vi "Request Channel.vi"(0 "Display State In":T2={"Hierarchy"=[], "File/Directory Path"=path "", "Relative File Paths"=[], "Hide Undefined Channels"=FALSE, "Static File Structure"=FALSE, "Filtering"={"Filtered Groups"=[], "Group Filter Mode"=enum."Exclude", "Group Filter Regex?"=FALSE, "Filtered Channels"=[], "Channel Filter Mode"=enum."Exclude", "Channel Filter Regex?"=FALSE, "Filter Time Start"=timestamp(0 s since 1904-01-01), "Filter Time End"=timestamp(0 s since 1904-01-01), "Time Filter Mode"=enum."Include", "Time Filter Enabled"=FALSE}, "File Contents Tree"=refnum, "Properties Table"=refnum, "Loading Indicator"=refnum}, 1 "Use Regular Expressions?":bool, 5 "Group Name":string, 7 "Channel Name":string, 9 "Container State":T5, 11 "error in (no error)":errorcluster) -> (4 "Display State Out":T2={"Hierarchy"=[], "File/Directory Path"=path "", "Relative File Paths"=[], "Hide Undefined Channels"=FALSE, "Static File Structure"=FALSE, "Filtering"={"Filtered Groups"=[], "Group Filter Mode"=enum."Exclude", "Group Filter Regex?"=FALSE, "Filtered Channels"=[], "Channel Filter Mode"=enum."Exclude", "Channel Filter Regex?"=FALSE, "Filter Time Start"=timestamp(0 s since 1904-01-01), "Filter Time End"=timestamp(0 s since 1904-01-01), "Time Filter Mode"=enum."Include", "Time Filter Enabled"=FALSE}, "File Contents Tree"=refnum, "Properties Table"=refnum, "Loading Indicator"=refnum}, 6 "Channel Data":T1[](array[typedef]), 15 "error out":errorcluster)   [LabVIEW 2017, in "XTree.xctl"]
doc: "Request one or more channels from the files currently represented in the tree. The Group Name and Channel Name inputs support regular expressions."
uses:
  <vilib>/addons/_NIFileIO/XTree/XTree.xctl
  <vilib>/_xctls/Container State.ctl
  <vilib>/addons/_NIFileIO/XTree/State.ctl
  <vilib>/addons/_NIFileIO/XTree/Controls/Filter Settings.ctl
  <vilib>/addons/_NIFileIO/XTree/Controls/Filter Mode.ctl
  <vilib>/addons/_NIFileIO/XTree/Controls/Tree Selection Data.ctl
  <vilib>/_xctls/XControlSupport.lvlib
panel:
  # "Add Controls & Indicators that form the parameters of the method here. Hook them to the connector pane. Do not delete the controls & indicators that are already hooked to the connector pane.\n \nTo setup the parameters  for this method, right click on this item in the Project Tree & select \"Configure Method...\"."
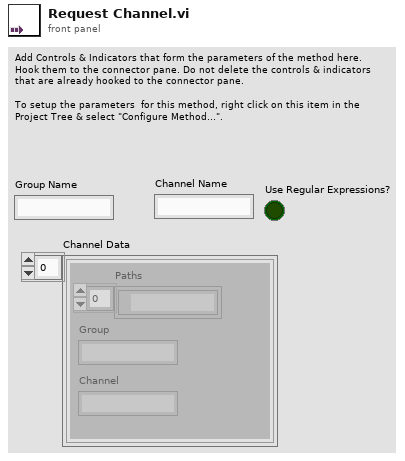
[diagram p1: front panel]
types:
  T1 = typedef "XTree.xctl/Tree Selection Data.ctl" = cluster{"Paths":path[], "Group":string, "Channel":string}
  T2 = typedef "XTree.xctl/State.ctl" = cluster{"Hierarchy":string[], "File/Directory Path":path, "Relative File Paths":string[], "Hide Undefined Channels":bool, "Static File Structure":bool, "Filtering":T3, "File Contents Tree":refnum<vi>, "Properties Table":refnum<vi>, "Loading Indicator":refnum<vi>}
  T3 = typedef "XTree.xctl/Filter Settings.ctl" = cluster{"Filtered Groups":string[], "Group Filter Mode":T4, "Group Filter Regex?":bool, "Filtered Channels":string[], "Channel Filter Mode":T4, "Channel Filter Regex?":bool, "Filter Time Start":timestamp, "Filter Time End":timestamp, "Time Filter Mode":T4, "Time Filter Enabled":bool}
  T4 = typedef "XTree.xctl/Filter Mode.ctl" = enum16{"Exclude", "Include"}
  T5 = typedef "XControlSupport.lvlib/Container State.ctl" = cluster{"Indicator?":bool, "Run Mode?":bool, " Refnum":refnum<vi>}
  T6 = enum16{"open", "open or create", "create or replace", "create", "open (read-only)"}
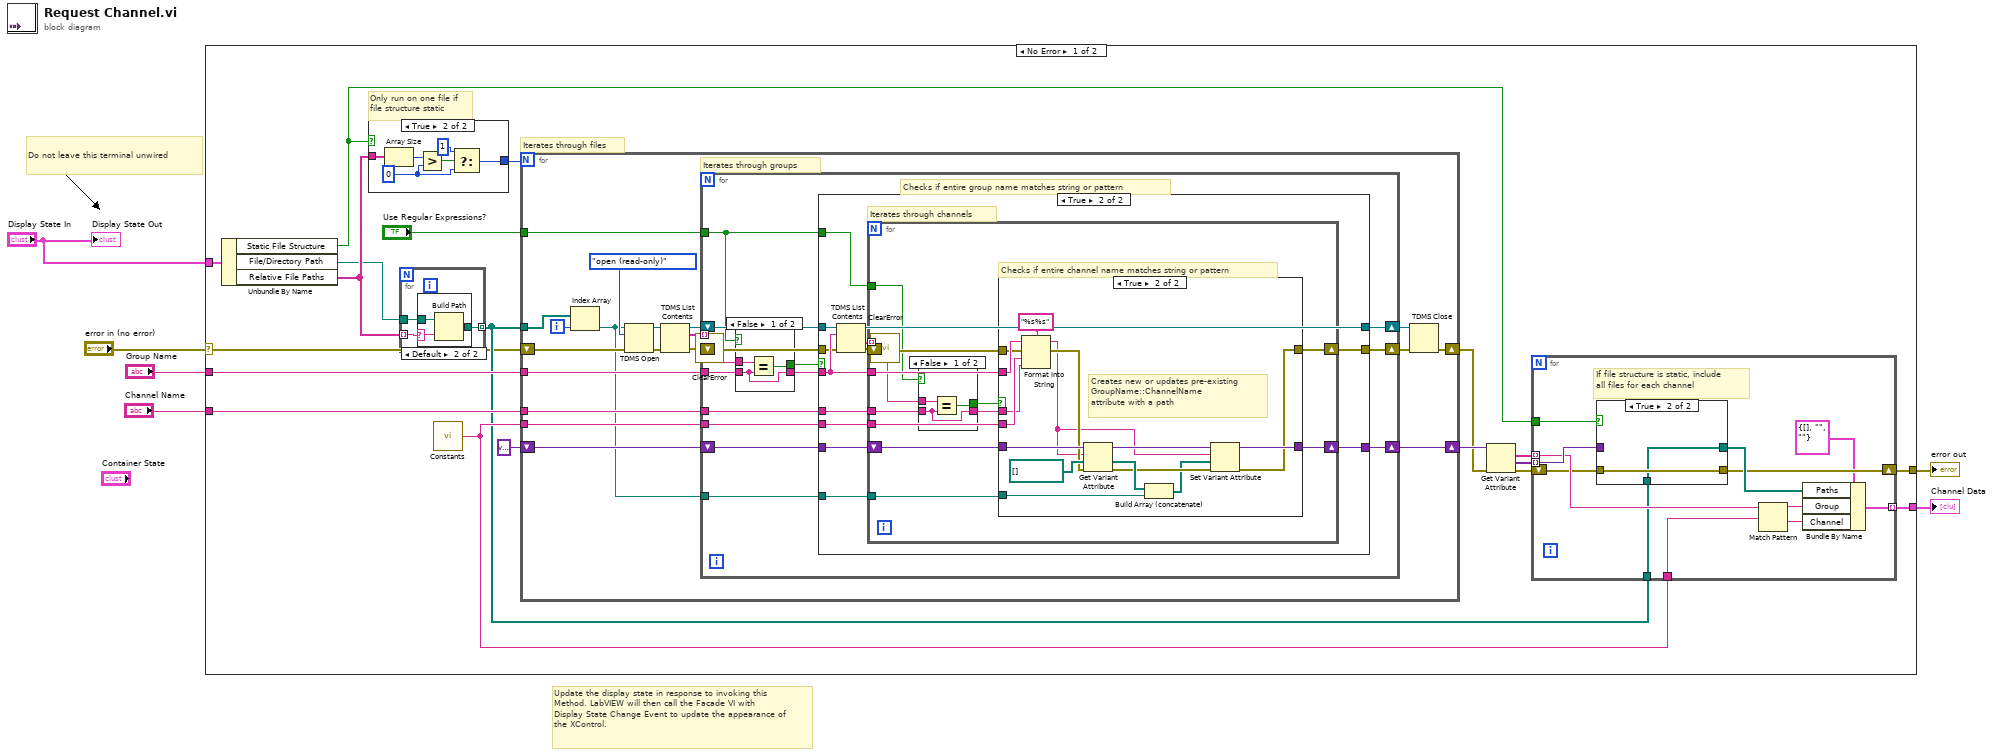
[diagram p0: block diagram]
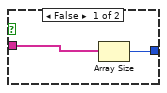
[diagram p3: hidden frame]
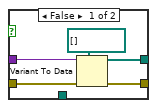
[diagram p4: hidden frame]
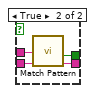
[diagram p5: hidden frame]
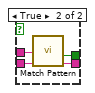
[diagram p7: hidden frame]
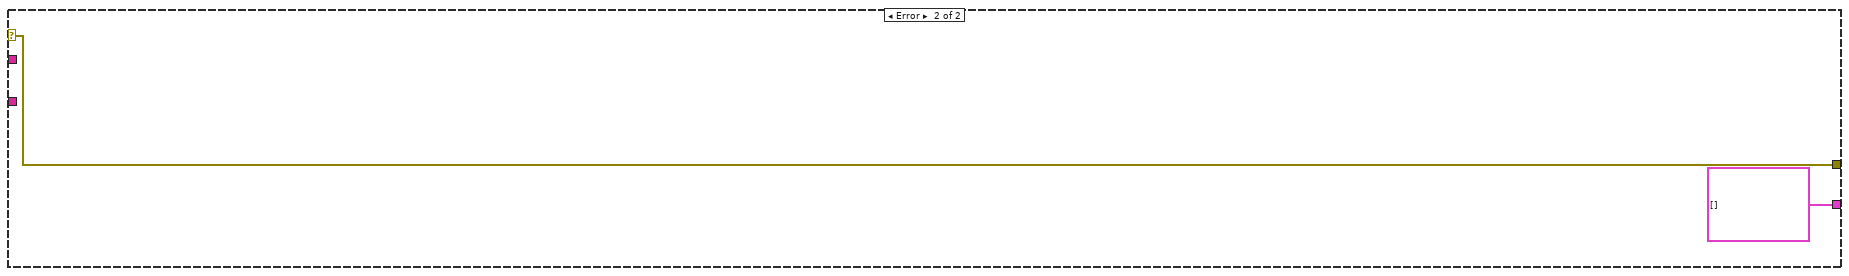
[diagram p9: hidden frame]
diagram:
  # "Do not leave this terminal unwired"
  # "Update the display state in response to invoking this Method. LabVIEW will then call the Facade VI with Display State Change Event to update the appearance of the XControl."
  n1 = case shown="No Error" "error in (no error)" {
    selector: "error in (no error)" -> [w7 w156]
    tunnel: "Display State In" -> [w25 _]
    tunnel: "Group Name" -> [w24 _]
    tunnel: "Channel Name" -> [w23 _]
    tunnel: [w17 T1[] []] -> w3
    tunnel: [w13 w156] -> w2
    frame No Error {
      # "Iterates through files"
      # "Only run on one file if file structure static"
      n2 = Unbundle By Name(w25) -> ("Static File Structure"=w12:bool, "File/Directory Path"=w8:path, "Relative File Paths"=w11:string[])
      n3 = case shown="True" w12 {
        tunnel: [w34 w35] -> w15
        tunnel: w11 -> [w33 w40]
        frame False {
          n4 = Array Size(array=w33) -> (size(s)=w34:i32)
        }
        frame True {
          w37 = 0 ("y")
          n5 = Array Size(array=w40) -> (size(s)=w39:i32)
          n6 = Greater?(x=w39, y=w37) -> (0:w38:bool)
          n7 = Select(t=1, s=w38, f=w37) -> (s? t:f=w35:i32)
        }
      }
      n8 = for {
        tunnel: w11 -> [w26] mode=indexing
        tunnel: w8 -> [w28]
        tunnel: [w27] -> w10 mode=indexing
        n9 = case shown="Default" w26 {
          selector: w26 -> [_ w30]
          tunnel: w28 -> [w29 w32]
          tunnel: [w29 w31] -> w27
          frame "" {
          }
          frame Default {
            n10 = Build Path(base path=w32, name or relative path=w30) -> (appended path=w31:path)
          }
        }
      }
      n11 = call <vilib>:"Constants.vi"() -> ("String Delimeter"=w16:string)  [unwired: 5 in]
      n12 = for {
        N: w15 -> [_]
        shift-right: [w79] -> w20
        shift-left: w7 -> [w65]
        tunnel: w24 -> [w74]
        tunnel: w23 -> [w72]
        tunnel: w16 -> [w67]
        shift-right: [w66] -> w21
        shift-left: variant ("variant") -> [w68]
        tunnel: w10 -> [w63]
        tunnel: "Use Regular Expressions?" -> [w64]
        i -> [w61]
        # "Iterates through groups"
        n13 = Index Array(array=w63, index=w61) -> (element=w62:path)
        n14 = TDMS Open(8:w65, 10:T6."open (read-only)" ("operation (0:open)"), 11:w62) -> (0:w77:errorcluster, 3:w76:refnum<k34>)  [unwired: 4 in]
        n15 = TDMS List Contents(4:w77, 7:w76) -> (0:w60:errorcluster, 2:w75:string[], 3:w73:refnum<k34>)  [unwired: 1 in, 1 out]
        n16 = call <vilib>:"ClearError.vi"("error in (no error)"=w60) -> ("error out"=w70:errorcluster)
        n17 = for {
          tunnel: w75 -> [w93] mode=indexing
          tunnel: w74 -> [w91]
          tunnel: w72 -> [w89]
          shift-right: [w88] -> w71
          shift-left: w73 -> [w92]
          shift-right: [w87] -> w69
          shift-left: w70 -> [w82]
          tunnel: w67 -> [w85]
          tunnel: w62 -> [w84]
          shift-right: [w83] -> w66
          shift-left: w68 -> [w86]
          tunnel: w64 -> [w80]
          # "Checks if entire group name matches string or pattern"
          n18 = case shown="False" w80 {
            tunnel: w93 -> [w96 w98]
            tunnel: w91 -> [w94 w100]
            tunnel: [w94 w99] -> w90
            tunnel: [w95 w97] -> w81
            frame False {
              n19 = Equal?(x=w96, y=w94) -> (x = y?=w95:bool)
            }
            frame True {
              n20 = call <vilib>:"Match Pattern.vi"("Pattern"=w100, "String in"=w98) -> ("String out"=w99:string, "Match?"=w97:bool)  [unwired: 8 in]
            }
          }
          n21 = case shown="True" w81 {
            tunnel: w90 -> [_ w114]
            tunnel: w92 -> [w103 w117]
            tunnel: w89 -> [_ w115]
            tunnel: [w103 w113] -> w88
            tunnel: w82 -> [w102 w112]
            tunnel: [w102 w110] -> w87
            tunnel: w86 -> [w101 w109]
            tunnel: w85 -> [_ w108]
            tunnel: w84 -> [_ w107]
            tunnel: [w101 w106] -> w83
            tunnel: w80 -> [_ w105]
            frame False {
            }
            frame True {
              # "Iterates through channels"
              n22 = TDMS List Contents(4:w112, 6:w114, 7:w117) -> (0:w104:errorcluster, 1:w116:string[], 3:w113:refnum<k34>)  [unwired: 1 out]
              n23 = call <vilib>:"ClearError.vi"("error in (no error)"=w104) -> ("error out"=w111:errorcluster)
              n24 = for {
                tunnel: w116 -> [w121] mode=indexing
                tunnel: w115 -> [w120]
                tunnel: w114 -> [w129]
                shift-right: [w128] -> w110
                shift-left: w111 -> [w123]
                tunnel: w108 -> [w126]
                tunnel: w107 -> [w125]
                shift-right: [w124] -> w106
                shift-left: w109 -> [w127]
                tunnel: w105 -> [w122]
                # "Checks if entire channel name matches string or pattern"
                n25 = case shown="False" w122 {
                  tunnel: w121 -> [w132 w134]
                  tunnel: w120 -> [w130 w136]
                  tunnel: [w130 w135] -> w118
                  tunnel: [w131 w133] -> w119
                  frame False {
                    n26 = Equal?(x=w132, y=w130) -> (x = y?=w131:bool)
                  }
                  frame True {
                    n27 = call <vilib>:"Match Pattern.vi"("Pattern"=w136, "String in"=w134) -> ("String out"=w135:string, "Match?"=w133:bool)  [unwired: 8 in]
                  }
                }
                n28 = case shown="True" w119 {
                  tunnel: w129 -> [_ w152]
                  tunnel: w123 -> [w138 w151]
                  tunnel: [w138 w142] -> w128
                  tunnel: w127 -> [w137 w154]
                  tunnel: w126 -> [_ w153]
                  tunnel: w125 -> [_ w144]
                  tunnel: [w137 w143] -> w124
                  tunnel: w118 -> [_ w139]
                  frame False {
                  }
                  frame True {
                    # "Creates new or updates pre-existing\nGroupName::ChannelName\nattribute with a path"
                    n29 = Format Into String(format string="%s%s", initial string=w152, error in=w151, w153, w139) -> (resulting string=w145:string, error out=w149:errorcluster)
                    n30 = Get Variant Attribute(Variant=w154, name=w145, default value (empty Variant)=path[] [], error in=w149) -> (duplicate Variant=w148:variant, value=w147:path[], error out=w146:errorcluster)  [unwired: 1 out]
                    n31 = Build Array (concatenate)(w147, w144) -> (w140:path[])
                    n32 = Set Variant Attribute(Variant=w148, name=w145, value=w140, error in=w146) -> (Variant out=w143:variant, error out=w142:errorcluster)  [unwired: 1 out]
                  }
                }
              }
            }
          }
        }
        n33 = TDMS Close(8:w69, 11:w71) -> (0:w79:errorcluster)  [unwired: 1 out]
      }
      n34 = Get Variant Attribute(Variant=w21, error in=w20) -> (names=w19:string[], values=w18:variant[], error out=w14:errorcluster)  [unwired: 2 in, 1 out]
      n35 = for {
        tunnel: w19 -> [w48] mode=indexing
        tunnel: w18 -> [w52] mode=indexing
        tunnel: [w47] -> w17 mode=indexing
        tunnel: w16 -> [w46]
        tunnel: w12 -> [w45]
        shift-right: [w43] -> w13
        shift-left: w14 -> [w44]
        tunnel: w10 -> [w42]
        # "If file structure is static, include all files for each channel"
        n36 = case shown="True" w45 {
          tunnel: w52 -> [w53 _]
          tunnel: [w56 w58] -> w51
          tunnel: w44 -> [w55 w59]
          tunnel: [w54 w59] -> w43
          tunnel: w42 -> [_ w58]
          frame False {
            n37 = Variant To Data(error in=w55, type=path[] [], Variant=w53) -> (data=w56:path[], error out=w54:errorcluster)
          }
          frame True {
          }
        }
        n38 = Match Pattern(string=w48, regular expression=w46) -> (before substring=w50:string, after substring=w49:string)  [unwired: 1 in, 2 out]
        n39 = Bundle By Name(cluster=T1 {"Paths"=[], "Group"="", "Channel"=""} ("Tree Selection Data"), "Paths"=w51, "Group"=w50, "Channel"=w49) -> (w47:T1)
      }
    }
    frame Error {
    }
  }
  "error out" <- w2
  "Channel Data" <- w3
  "Display State Out" <- "Display State In"
